vi "ui_ClientSrv Query Access Password.vi"(7 "access level":T1=enum."operator", 11 "test error in":errorcluster) -> (4 "OKed?":bool, 8 "access reason out":string, 15 "access password out":string)   [LabVIEW 2012]
doc: "This dialog allows entry of the password required to acquire the specified access level on the currently connected server and optionally specify a reason to other users."
uses:
  typedefs/t_ClientSrv Access Levels.ctl
  typedefs/t_ClientSrv Query Access Password States.ctl
panel:
  in  "access reason":string
  out "access status":string
  in  "access password":string
  in  "cancel":bool
  in  "OK":bool
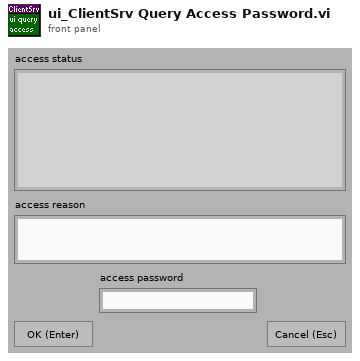
[diagram p1: front panel]
types:
  T1 = typedef "t_ClientSrv Access Levels.ctl" = enum16{"observer", "operator", "local"}
  T2 = typedef "t_ClientSrv Query Access Password States.ctl" = enum16{"empty queue", "do OK", "initialize", "stop"}
  T3 = typedef "eventvkey.ctl" = enum16{"ASCII", "Enter", "Return", "Shift", "Ctrl", "Alt", "Cmd", "Opt", "Caps", "NumLock", "Clear", "Break", "Up", "Down", "Left", "Right", "Insert", "Delete", "Home", "End", "PageUp", "PageDown", "Escape", "Help", "Pause", "ScrollLock", "F1", "F2", "F3", "F4", "F5", "F6", "F7", "F8", "F9", "F10", "F11", "F12", "F13", "F14", "F15", "F16", "F17", "F18", "F19", "F20", "F21", "F22", "F23", "F24", "Play", "VolumeUp", "VolumeDown", "Mute", "Two Byte Char"}
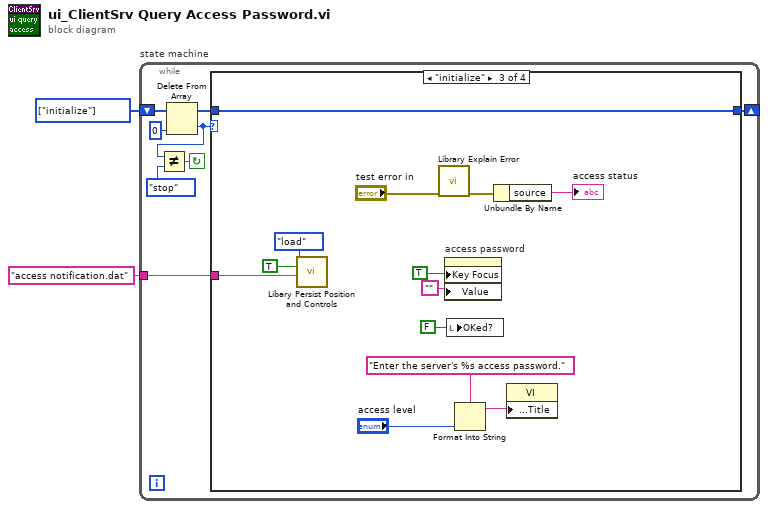
[diagram p0: block diagram]
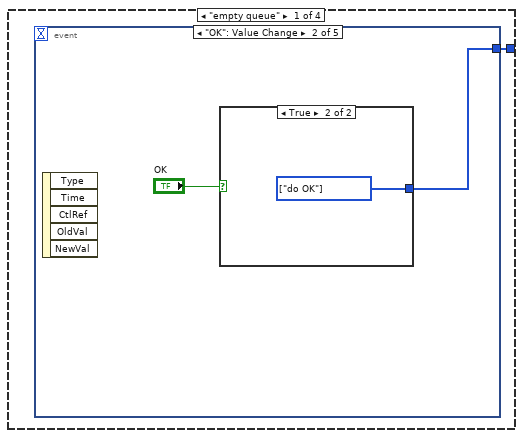
[diagram p2: hidden frame]
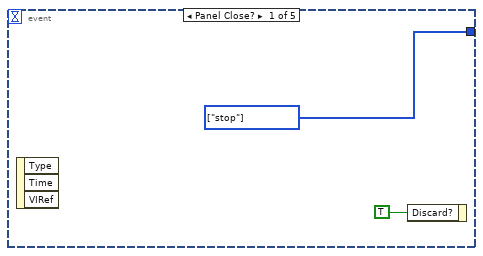
[diagram p3: hidden frame]
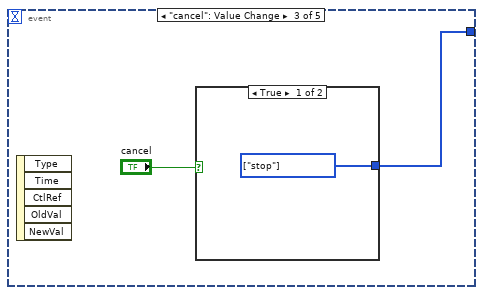
[diagram p5: hidden frame]
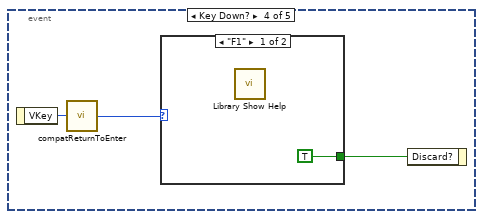
[diagram p7: hidden frame]
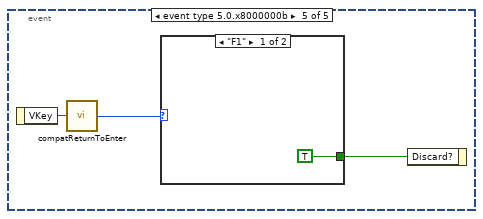
[diagram p9: hidden frame]
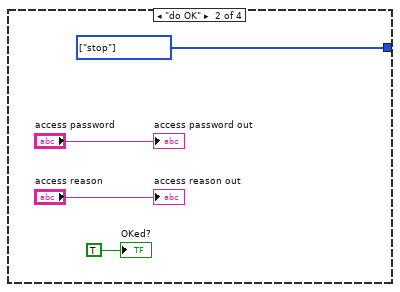
[diagram p11: hidden frame]
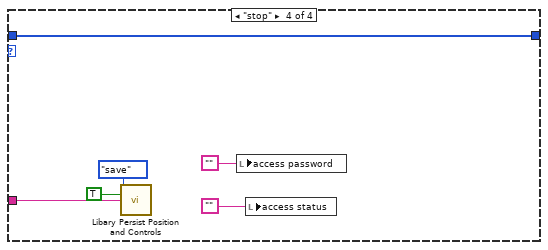
[diagram p12: hidden frame]
diagram:
  w2 = T2[] [enum."initialize"] items=["empty queue", "do OK", "initialize", "stop"] ("Array Constant")
  n1 = while "state machine" {
    shift-left: w2 -> [w7]
    shift-right: [w10] -> _
    tunnel: "access notification.dat" ("filename (<window title>.dat)") -> [w3]
    stop <- w9 continue-if-true
    n2 = Delete From Array(array=w7, index=0) -> (deleted portion=w5:T2, array with subset deleted=w6:T2[])  [unwired: 1 in]
    n3 = Not Equal?(x=w5, y=t_ClientSrv_Query_Access_Password_States."stop" ("states")) -> (x != y?=w9:bool)
    n4 = case "Case" shown="\"initialize\"" w5 {
      tunnel: [w11 w29 w44 w50] -> w10
      tunnel: w6 -> [_ _ w44 w50]
      tunnel: w3 -> [_ _ w34 w45]
      frame "empty queue" {
        n5 = event shown="[1] \"OK\": Value Change" {
          selector: _ -> [_ _ _ _ _]
          dyn-events: _ -> [_ _ _ _ _]
          timeout: _ -> [_ _ _ _ _]
          tunnel: [w13 w15 w18 _ _] -> w11
          event Panel Close? {
            w13 = T2[] [enum."stop"] items=["empty queue", "do OK", "initialize", "stop"] ("Array Constant")
            n6 = event-data() -> ()  [unwired: 1 in, 3 out]
            n7 = event-data("Discard?"=TRUE) -> ()  [unwired: 1 in, 1 out]
          }
          event "OK": Value Change {
            n8 = event-data() -> ()  [unwired: 1 in, 5 out]
            n9 = case shown="True" "OK" {
              tunnel: [_ w16] -> w15
              frame False {
              }
              frame True {
                w16 = T2[] [enum."do OK"] items=["empty queue", "do OK", "initialize", "stop"] ("Array Constant")
              }
            }
          }
          event "cancel": Value Change {
            n10 = event-data() -> ()  [unwired: 1 in, 5 out]
            n11 = case shown="True" "cancel" {
              tunnel: [w19 _] -> w18
              frame True {
                w19 = T2[] [enum."stop"] items=["empty queue", "do OK", "initialize", "stop"] ("Array Constant")
              }
              frame False {
              }
            }
          }
          event Key Down? {
            n12 = event-data() -> ("VKey"=w20:T3)  [unwired: 1 in]
            n13 = call <vilib>:"compatReturnToEnter.vi"("VKey"=w20) -> ("VKey"=w22:T3)
            n14 = case shown="\"F1\"" w22 {
              tunnel: [TRUE ("Discard?") _] -> w21
              frame "F1" {
                n15 = call "Library Show Help.vi"() -> ()  [unwired: 1 in]
              }
              frame Default {
              }
            }
            n16 = event-data("Discard?"=w21) -> ()  [unwired: 1 in, 1 out]
          }
          event event type 5.0.x8000000b {
            n17 = event-data() -> ("VKey"=w24:T3)  [unwired: 1 in]
            n18 = call <vilib>:"compatReturnToEnter.vi"("VKey"=w24) -> ("VKey"=w26:T3)
            n19 = case shown="\"F1\"" w26 {
              tunnel: [TRUE ("Discard?") _] -> w25
              frame "F1" {
              }
              frame Default {
              }
            }
            n20 = event-data("Discard?"=w25) -> ()  [unwired: 1 in, 1 out]
          }
        }
      }
      frame "do OK" {
        w29 = T2[] [enum."stop"] items=["empty queue", "do OK", "initialize", "stop"] ("Array Constant")
        "OKed?" <- TRUE ("OKed?")
        "access password out" <- "access password"
        "access reason out" <- "access reason"
      }
      frame "initialize" {
        n21 = call "Libary Persist Position and Controls.vi"("action"=enum16{"save", "load"}."load", "do not persist bounds (false)"=TRUE, "filename (<window title hash>.dat)"=w34) -> ()  [unwired: 11 in, 2 out]
        n22 = call "Library Explain Error.vi"("error in (no error)"="test error in") -> ("explained error"=w32:errorcluster)  [unwired: 14 in]
        n23 = property on="access password" class="Str"("Key Focus"=TRUE, "Value"="" ("machine name")) -> ()  [unwired: 2 in, 2 out]
        n24 = local write "OKed?"(FALSE ("OKed?")) -> ()
        n25 = Format Into String(format string="Enter the server's %s access password.", "access level") -> (resulting string=w37:string)  [unwired: 2 in, 1 out]
        n26 = Unbundle By Name(w32) -> ("source"=→"access status":string)
        n27 = property class="VI"("Front Panel Window:Title"=w37) -> ()  [unwired: 2 in, 2 out]
      }
      frame "stop" {
        n28 = call "Libary Persist Position and Controls.vi"("action"=enum16{"save", "load"}."save", "do not persist bounds (false)"=TRUE, "filename (<window title hash>.dat)"=w45) -> ()  [unwired: 11 in, 2 out]
        n29 = local write "access password"("") -> ()
        n30 = local write "access status"("") -> ()
      }
    }
  }
